vi "TextDocument_GetCommonStyles.vi"(8 "error in":errorcluster, 11 "TextDocument in":refnum<k24>) -> (0 "error out":errorcluster, 2 "Common Styles":string[](array[string]), 3 "TextDocument out":refnum<k24>)   [LabVIEW 2009]
uses:
  C:/Projets/LAVAG/OpenOfficeRGT/AODL/DLLs/AODL.dll
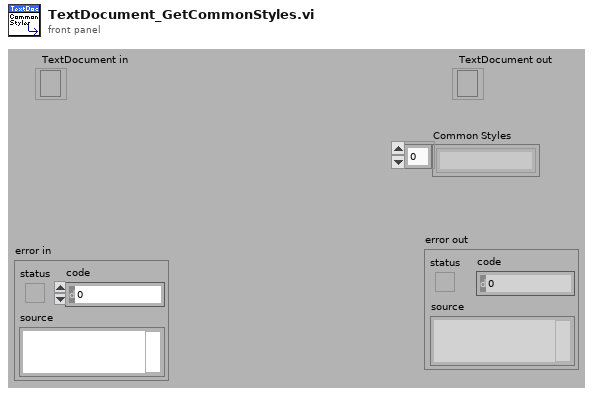
[diagram p1: front panel]
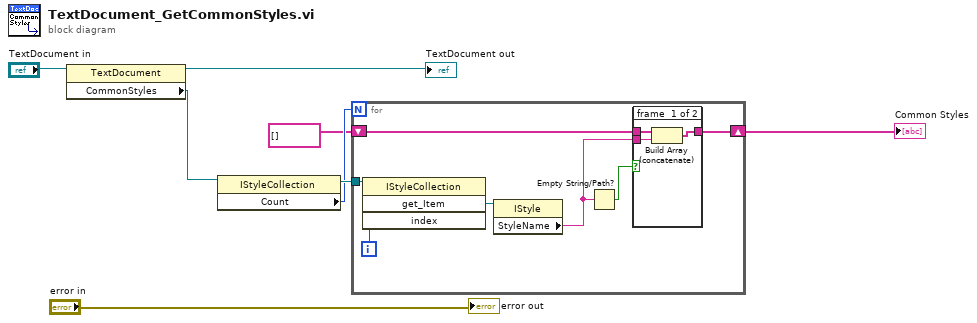
[diagram p0: block diagram]
diagram:
  n1 = property class="TextDocument"(reference="TextDocument in") -> (reference out=→"TextDocument out":refnum<k24>, "CommonStyles"=w6:refnum<k24>)  [unwired: 1 in, 1 out]
  n2 = property class="IStyleCollection"(reference=w6) -> (reference out=w5:refnum<k24>, "Count"=w4:i32)  [unwired: 1 in, 1 out]
  n3 = for {
    N: w4 -> [_]
    tunnel: w5 -> [w15]
    shift-right: [w10] -> w1
    shift-left: string[] [] -> [w11]
    i -> [w14]
    n4 = invoke class="IStyleCollection" method="get_Item"(reference=w15, "index"=w14) -> ("get_Item"=w13:refnum<k24>)  [unwired: 2 in, 3 out]
    n5 = property class="IStyle"(reference=w13) -> ("StyleName"=w9:string)  [unwired: 1 in, 2 out]
    n6 = Empty String/Path?(string/path=w9) -> (empty?=w12:bool)
    n7 = case shown="False" w12 {
      tunnel: w11 -> [w18 w19]
      tunnel: [w17 w19] -> w10
      tunnel: w9 -> [w16 _]
      frame #0 {
        n8 = Build Array (concatenate)(w18, w16) -> (w17:string[])
      }
      frame #1 {
      }
    }
  }
  "Common Styles" <- w1
  "error out" <- "error in"
